vi "Finish.vi"   [LabVIEW 2014]
doc: "This VI is called just before exiting. It is expected to close I/O refnum, save collected data, etc."
uses:
  <vilib>/Rock Robotics/WPI/Joystick/WPI_JoystickGetSetRefNum.vi
  <vilib>/Rock Robotics/WPI/RobotDrive/WPI_RobotDriveGetSetRefNum.vi
types:
  T1 = typedef "WPI_MotorControlDeviceRef.ctl" = cluster{"DeviceStatus":errorcluster, "Type":T2, "PWM":cluster{"Controller":T3, "PWM Channel":T4, "DeadBand":T5}, "CAN":cluster{"Device Number":u8, "Control Mode":T6, "Semaphore":T7, "Max Vout":dbl, "TalonSRX Control Mode":T8}, "Invert":bool, "TransformRef":T9, "InvTransformRef":T9}
  T2 = typedef "WPI_MotorControlType.ctl" = enum16{"PWM", "CAN", "CANTalonSRX"}
  T3 = typedef "FPGA_TypedefDigitalModule.ctl" = enum16{"Controller 1"}
  T4 = typedef "FPGA_DIOPWMChannel.ctl" = enum8{"PWM 0", "PWM 1", "PWM 2", "PWM 3", "PWM 4", "PWM 5", "PWM 6", "PWM 7", "PWM 8", "PWM 9", "PWM MXP 0", "PWM MXP 1", "PWM MXP 2", "PWM MXP 3", "PWM MXP 4", "PWM MXP 5", "PWM MXP 6", "PWM MXP 7", "PWM MXP 8", "PWM MXP 9", "Invalid"}
  T5 = typedef "WPI_PWMDeadband.ctl" = cluster{"Name":string, "maxPositivePwm":i32, "minPositivePwm":i32, "centerPwm":i32, "maxNegativePwm":i32, "minNegativePwm":i32, "angularRange":u16}
  T6 = typedef "WPI_CANJaguar_ControlMode.ctl" = enum8{"Percent VBus", "Current", "Speed", "Position", "Voltage"}
  T7 = typedef "Semaphore RefNum" = refnum<k1>
  T8 = typedef "WPI_CANTalonSRX_APIControlMode.ctl" = enum8{"Percent VBus", "Speed", "Position", "Slave", "Unchanged / Invalid"}
  T9 = typedef "WPI_PWMTransform_ConPane.ctl" = refnum<vi>
  T10 = typedef "WPI_JoystickDevRef.ctl" = cluster{"Device":T11}
  T11 = typedef "WPI_JoystickDeviceEnum.ctl" = enum16{"USB 0", "USB 1", "USB 2", "USB 3", "USB 4", "USB 5"}
  T12 = typedef "WPI_RobotDriveDevRef.ctl" = cluster{"DevStatus":errorcluster, "Motors[]":T1[], "Square Inputs":bool, "Max Output":dbl}
  T13 = typedef "WPI_DigitalInputDevRef.ctl" = cluster{"DevStatus":errorcluster, "DIO Channel":T14, "Controller":T3}
  T14 = typedef "FPGA_DIOChannel.ctl" = enum8{"DIO 0", "DIO 1", "DIO 2", "DIO 3", "DIO 4", "DIO 5", "DIO 6", "DIO 7", "DIO 8", "DIO 9", "DIO MXP 0", "DIO MXP 1", "DIO MXP 2", "DIO MXP 3", "DIO MXP 4", "DIO MXP 5", "DIO MXP 6", "DIO MXP 7", "DIO MXP 8", "DIO MXP 9", "DIO MXP 10", "DIO MXP 11", "DIO MXP 12", "DIO MXP 13", "DIO MXP 14", "DIO MXP 15", "Invalid"}
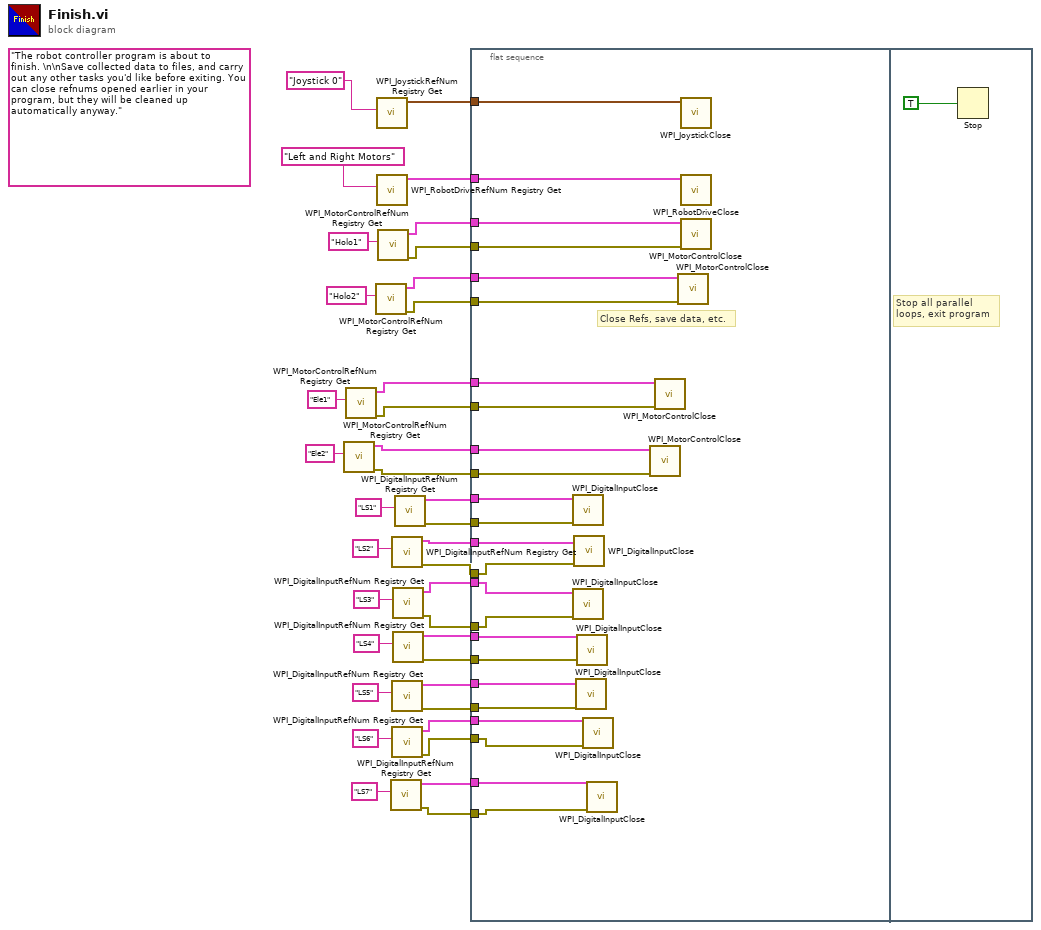
[diagram p0: block diagram]
diagram:
  (unwired) "The robot controller program is about to finish. \n\nSave collected data to files, and carry out any other tasks you'd like before exiting. You can close refnums opened earlier in your program, but they will be cleaned up automatically anyway."
  n1 = call <vilib>:"WPI_MotorControlRefNum Registry Get.vi"("refnum name"="Ele2") -> ("error out"=w22:errorcluster, "MotorControlDevRef"=w23:T1)  [unwired: 9 in]
  n2 = call <vilib>:"WPI_MotorControlRefNum Registry Get.vi"("refnum name"="Ele1") -> ("error out"=w24:errorcluster, "MotorControlDevRef"=w25:T1)  [unwired: 9 in]
  n3 = call <vilib>:"WPI_MotorControlRefNum Registry Get.vi"("refnum name"="Holo2") -> ("error out"=w32:errorcluster, "MotorControlDevRef"=w33:T1)  [unwired: 9 in]
  n4 = call <vilib>:"WPI_JoystickRefNum Registry Get.vi"("refnum name"="Joystick 0") -> ("JoystickDevRef"=w34:T10)  [unwired: 1 in, 9 out]
  n5 = call <vilib>:"WPI_RobotDriveRefNum Registry Get.vi"("refnum name"="Left and Right Motors") -> ("RobotDriveDevRef"=w35:T12)  [unwired: 1 in, 9 out]
  n6 = call <vilib>:"WPI_MotorControlRefNum Registry Get.vi"("refnum name"="Holo1") -> ("error out"=w30:errorcluster, "MotorControlDevRef"=w31:T1)  [unwired: 9 in]
  n7 = call <vilib>:"WPI_DigitalInputRefNum Registry Get.vi"("refnum name"="LS7") -> ("error out"=w2:errorcluster, "DigitalInputDevRef"=w1:T13)  [unwired: 9 in]
  n8 = call <vilib>:"WPI_DigitalInputRefNum Registry Get.vi"("refnum name"="LS2") -> ("error out"=w12:errorcluster, "DigitalInputDevRef"=w11:T13)  [unwired: 9 in]
  n9 = call <vilib>:"WPI_DigitalInputRefNum Registry Get.vi"("refnum name"="LS5") -> ("error out"=w6:errorcluster, "DigitalInputDevRef"=w5:T13)  [unwired: 9 in]
  n10 = call <vilib>:"WPI_DigitalInputRefNum Registry Get.vi"("refnum name"="LS6") -> ("error out"=w4:errorcluster, "DigitalInputDevRef"=w3:T13)  [unwired: 9 in]
  n11 = call <vilib>:"WPI_DigitalInputRefNum Registry Get.vi"("refnum name"="LS3") -> ("error out"=w10:errorcluster, "DigitalInputDevRef"=w9:T13)  [unwired: 9 in]
  n12 = call <vilib>:"WPI_DigitalInputRefNum Registry Get.vi"("refnum name"="LS4") -> ("error out"=w8:errorcluster, "DigitalInputDevRef"=w7:T13)  [unwired: 9 in]
  n13 = call <vilib>:"WPI_DigitalInputRefNum Registry Get.vi"("refnum name"="LS1") -> ("error out"=w14:errorcluster, "DigitalInputDevRef"=w13:T13)  [unwired: 9 in]
  n14 = flat-sequence {
    tunnel: w35 -> [w61]
    tunnel: w34 -> [w60]
    tunnel: w33 -> [w59]
    tunnel: w32 -> [w58]
    tunnel: w31 -> [w57]
    tunnel: w30 -> [w56]
    tunnel: w25 -> [w55]
    tunnel: w24 -> [w54]
    tunnel: w23 -> [w53]
    tunnel: w22 -> [w52]
    tunnel: w14 -> [w50]
    tunnel: w13 -> [w51]
    tunnel: w12 -> [w48]
    tunnel: w11 -> [w49]
    tunnel: w10 -> [w46]
    tunnel: w9 -> [w47]
    tunnel: w8 -> [w44]
    tunnel: w7 -> [w45]
    tunnel: w6 -> [w42]
    tunnel: w5 -> [w43]
    tunnel: w4 -> [w40]
    tunnel: w3 -> [w41]
    tunnel: w2 -> [w38]
    tunnel: w1 -> [w39]
    frame #0 {
      # "Close Refs, save data, etc."
      n15 = call <vilib>:"WPI_DigitalInputClose.vi"("error in (no error)"=w50, "DigitalInputDevRef"=w51) -> ()  [unwired: 9 in, 1 out]
      n16 = call <vilib>:"WPI_DigitalInputClose.vi"("error in (no error)"=w46, "DigitalInputDevRef"=w47) -> ()  [unwired: 9 in, 1 out]
      n17 = call <vilib>:"WPI_DigitalInputClose.vi"("error in (no error)"=w48, "DigitalInputDevRef"=w49) -> ()  [unwired: 9 in, 1 out]
      n18 = call <vilib>:"WPI_DigitalInputClose.vi"("error in (no error)"=w42, "DigitalInputDevRef"=w43) -> ()  [unwired: 9 in, 1 out]
      n19 = call <vilib>:"WPI_DigitalInputClose.vi"("error in (no error)"=w44, "DigitalInputDevRef"=w45) -> ()  [unwired: 9 in, 1 out]
      n20 = call <vilib>:"WPI_DigitalInputClose.vi"("error in (no error)"=w40, "DigitalInputDevRef"=w41) -> ()  [unwired: 9 in, 1 out]
      n21 = call <vilib>:"WPI_DigitalInputClose.vi"("error in (no error)"=w38, "DigitalInputDevRef"=w39) -> ()  [unwired: 9 in, 1 out]
      n22 = call <vilib>:"WPI_MotorControlClose.vi"("error in (no error)"=w52, "MotorControlDevRef"=w53) -> ()  [unwired: 9 in, 1 out]
      n23 = call <vilib>:"WPI_MotorControlClose.vi"("error in (no error)"=w54, "MotorControlDevRef"=w55) -> ()  [unwired: 9 in, 1 out]
      n24 = call <vilib>:"WPI_MotorControlClose.vi"("error in (no error)"=w58, "MotorControlDevRef"=w59) -> ()  [unwired: 9 in, 1 out]
      n25 = call <vilib>:"WPI_JoystickClose.vi"("JoystickDevRef"=w60) -> ()  [unwired: 11 out]
      n26 = call <vilib>:"WPI_RobotDriveClose.vi"("RobotDriveDevRef"=w61) -> ()  [unwired: 1 in, 10 out]
      n27 = call <vilib>:"WPI_MotorControlClose.vi"("error in (no error)"=w56, "MotorControlDevRef"=w57) -> ()  [unwired: 9 in, 1 out]
    }
    frame #1 {
      # "Stop all parallel\nloops, exit program"
      n28 = Stop(stop? (T)=TRUE ("Quit")) -> ()
    }
  }
